vi "Basic Commands.vi"(0 ".NET Refnum in":refnum<k24>, 1 "Database":string, 2 "Database Command":T1, 3 "Query":bool, 5 "SQL Command":string, 7 "Table":string, 9 "Column List":string[](array[string]), 11 "error in (no error)":errorcluster, 12 "Values":string[](array[string]), 13 "Condition":string) -> (4 "Data Array":string[][](array[string]), 6 "SQL Command out":string, 15 "error out":errorcluster)   [LabVIEW 2017, in "VIs to Interface LabVIEW and MySQL dotNET Connector.lvlib"]
doc: "All commands require Database and Table be wired\n\nInsert\nRequires: Columns, Values\n\nUpdate\nRequires: Columns, Values, Condition\n\nSelect All\nRequires: Nothing \n\nDelete Entry\nRequires: Condition\n\nDrop Table\nRequires: Nothing\n\nSQL Command\nRequires: SQL Command\n\nSelect\nRequires: Condition\n\nGet Column Info\nRequires: Nothing"
uses:
  VIs to Interface LabVIEW and MySQL dotNET Connector.lvlib
  Controls/Database Command.ctl
  MySql.Data
panel:
  # "All commands require Database and Table be wired\n\nInsert\nRequires: Columns, Values\n\nUpdate\nRequires: Columns, Values, Condition\n\nSelect All\nRequires: Nothing \n\nDelete Entry\nRequires: Condition\n\nDrop Table\nRequires: Nothing\n\nSQL Command\nRequires: SQL Command\n\nSelect\nRequires: Condition\n\nGet Column Info\nRequires: Nothing"
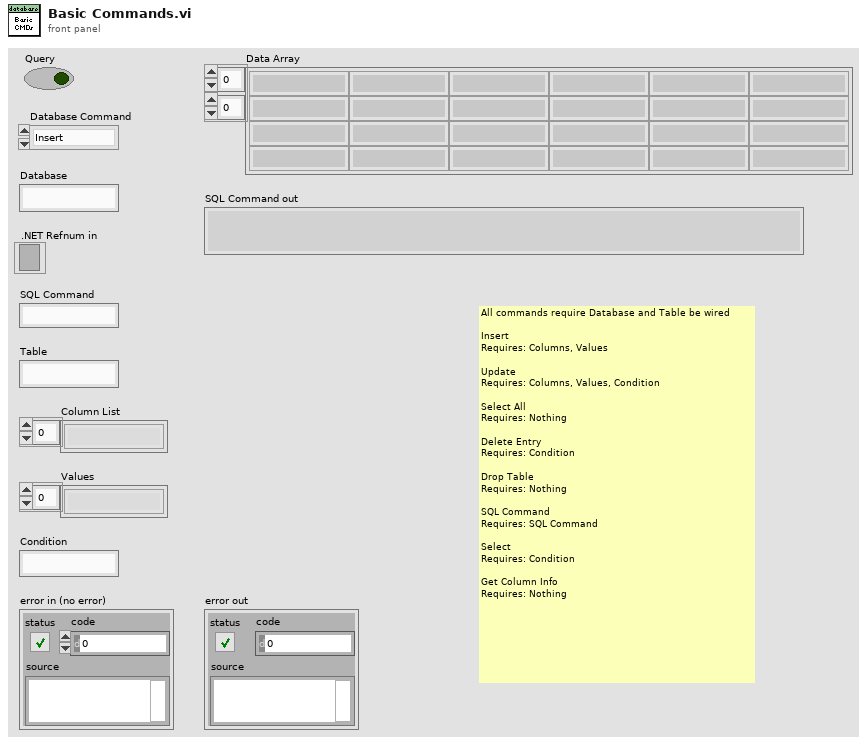
[diagram p1: front panel]
types:
  T1 = typedef "VIs to Interface LabVIEW and MySQL dotNET Connector.lvlib/Database Command.ctl" = enum16{"Insert", "Update", "Select All", "Delete Entry", "Drop Table", "SQL Command", "Select", "Get Column Info", "Select Column"}
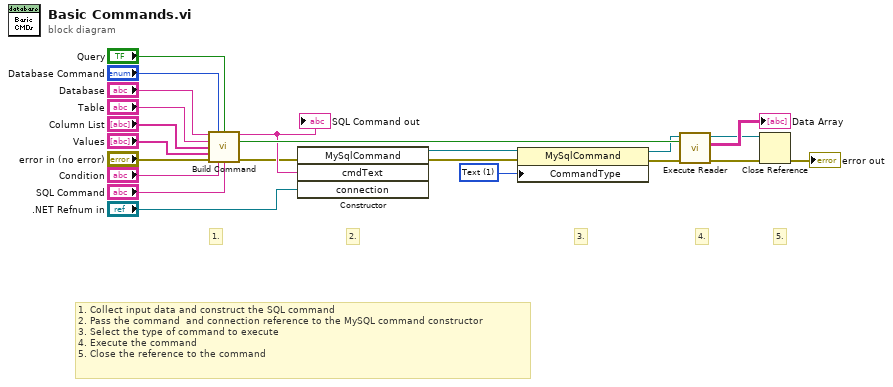
[diagram p0: block diagram]
diagram:
  w1 = 1 items=["Text"=1, "StoredProcedure"=4, "TableDirect"=512] ("CommandType")
  # "1. Collect input data and construct the SQL command\n2. Pass the command  and connection reference to the MySQL command constructor\n3. Select the type of command to execute\n4. Execute the command \n5. Close the reference to the command"
  # "5."
  # "4."
  # "3."
  # "2."
  # "1."
  n1 = call "Build Command.vi"("Database"="Database", "Database Command"="Database Command", "Query"="Query", "Table"="Table", "Column List"="Column List", "Values"="Values", "error in (no error)"="error in (no error)", "Condition"="Condition", "SQL Command in"="SQL Command") -> ("SQL Command out"=w19:string, "Query?"=w22:bool, "error out"=w18:errorcluster)  [unwired: 4 in]
  "SQL Command out" <- w19
  n2 = constructor class="MySqlCommand"(error in=w18, "cmdText"=w19, "connection"=".NET Refnum in") -> (reference out=w2:refnum<k24>, error out=w3:errorcluster)  [unwired: 2 in, 3 out]
  n3 = property class="MySqlCommand"(reference=w2, error in=w3, "CommandType"=w1) -> (reference out=w5:refnum<k24>, error out=w4:errorcluster)
  n4 = call "Execute Reader.vi"("error in (no error)"=w4, "Query?"=w22, ".NET Refnum in"=w5) -> ("error out"=w7:errorcluster, "Data"=→"Data Array":string[][], ".NET Refnum out"=w6:refnum<k24>)  [unwired: 6 in]
  n5 = Close Reference(reference=w6, error in (no error)=w7) -> (error out=→"error out":errorcluster)
